vi "PowerConversion.vi"() -> ()   [LabVIEW 2017, in "HMILibrary.lvlib"]
uses:
  HMILibrary.lvlib
  <vilib>/Platform/TimedLoop/XDataNode/timing_clust.ctl
  <vilib>/Platform/TimedLoop/XDataNode/nitl_modes.ctl
  <vilib>/Platform/TimedLoop/XDataNode/wakeup.ctl
  <vilib>/platform/TimedLoop/XDataNode/XDataNode.xnode
  <vilib>/express/express arith-compare/Formula/XNode/ExpressFormulaBlockNode.xnode
  <vilib>/Platform/TimedLoop/XDataNode/XDNodeRunTimeDep.lvlib
panel:
  out "P_1":dbl
  out "T_1":dbl
  out "P_2":dbl
  out "T_2":dbl
  out "P_3":dbl
  out "T_3":dbl
  out "P_4":dbl
  out "T_4":dbl
  out "P_5":dbl
  out "T_5":dbl
  out "P_6":dbl
  out "T_6":dbl
  out "R_P_4":dbl
  out "R_T_4":dbl
  out "h_4":dbl
  out "R_P_5":dbl
  out "R_T_5":dbl
  out "h_5":dbl
  out "R_P_6":dbl
  out "R_T_6":dbl
  out "h_6":dbl
  out "R_P_1":dbl
  out "R_T_1":dbl
  out "h_1":dbl
  in  "Compression Ratio":dbl=19.6
  in  "Incoming Air Temp":dbl=298.0
  in  "HPT Expansion Ratio":dbl=3.77
  in  "Incoming Air Pressure":dbl=101325.0
  in  "LPT Expansion Ratio":dbl=5.13
  in  "Compressor Efficiency":dbl=0.7
  in  "HPT Efficiency":dbl=0.8
  in  "LPT Efficiency":dbl=0.8
  in  "HPT Work Output":dbl=1000000.0
  in  "LPT Work Output":dbl=137940000.0
  in  "Pressure Drop in HX 1st pass":dbl
  in  "Pressure Drop in HX 2nd pass":dbl
  in  "Mass Flowrate":dbl=418.0
  in  "Lower Operating Pressure":dbl=7093.0
  in  "Pinch Point Temp Difference":dbl=15.0
  in  "Turbine Efficiency":dbl=0.95
  in  "Pump Efficiency":dbl=0.95
  in  "Upper Operating Pressure":dbl=6154480.5
  in  "stop":bool
  # "Power Conversion System"
  # "Brayton Cycle"
  # "Rankine Cycle"
  # "HRSG"
  # "Compressor"
  # "HPT"
  # "LPT"
  # "ST"
  # "Primary Heat\nExchanger"
  # "Condenser"
  # "Pump"
  # "Temperatures in K\nPressures in Pa"
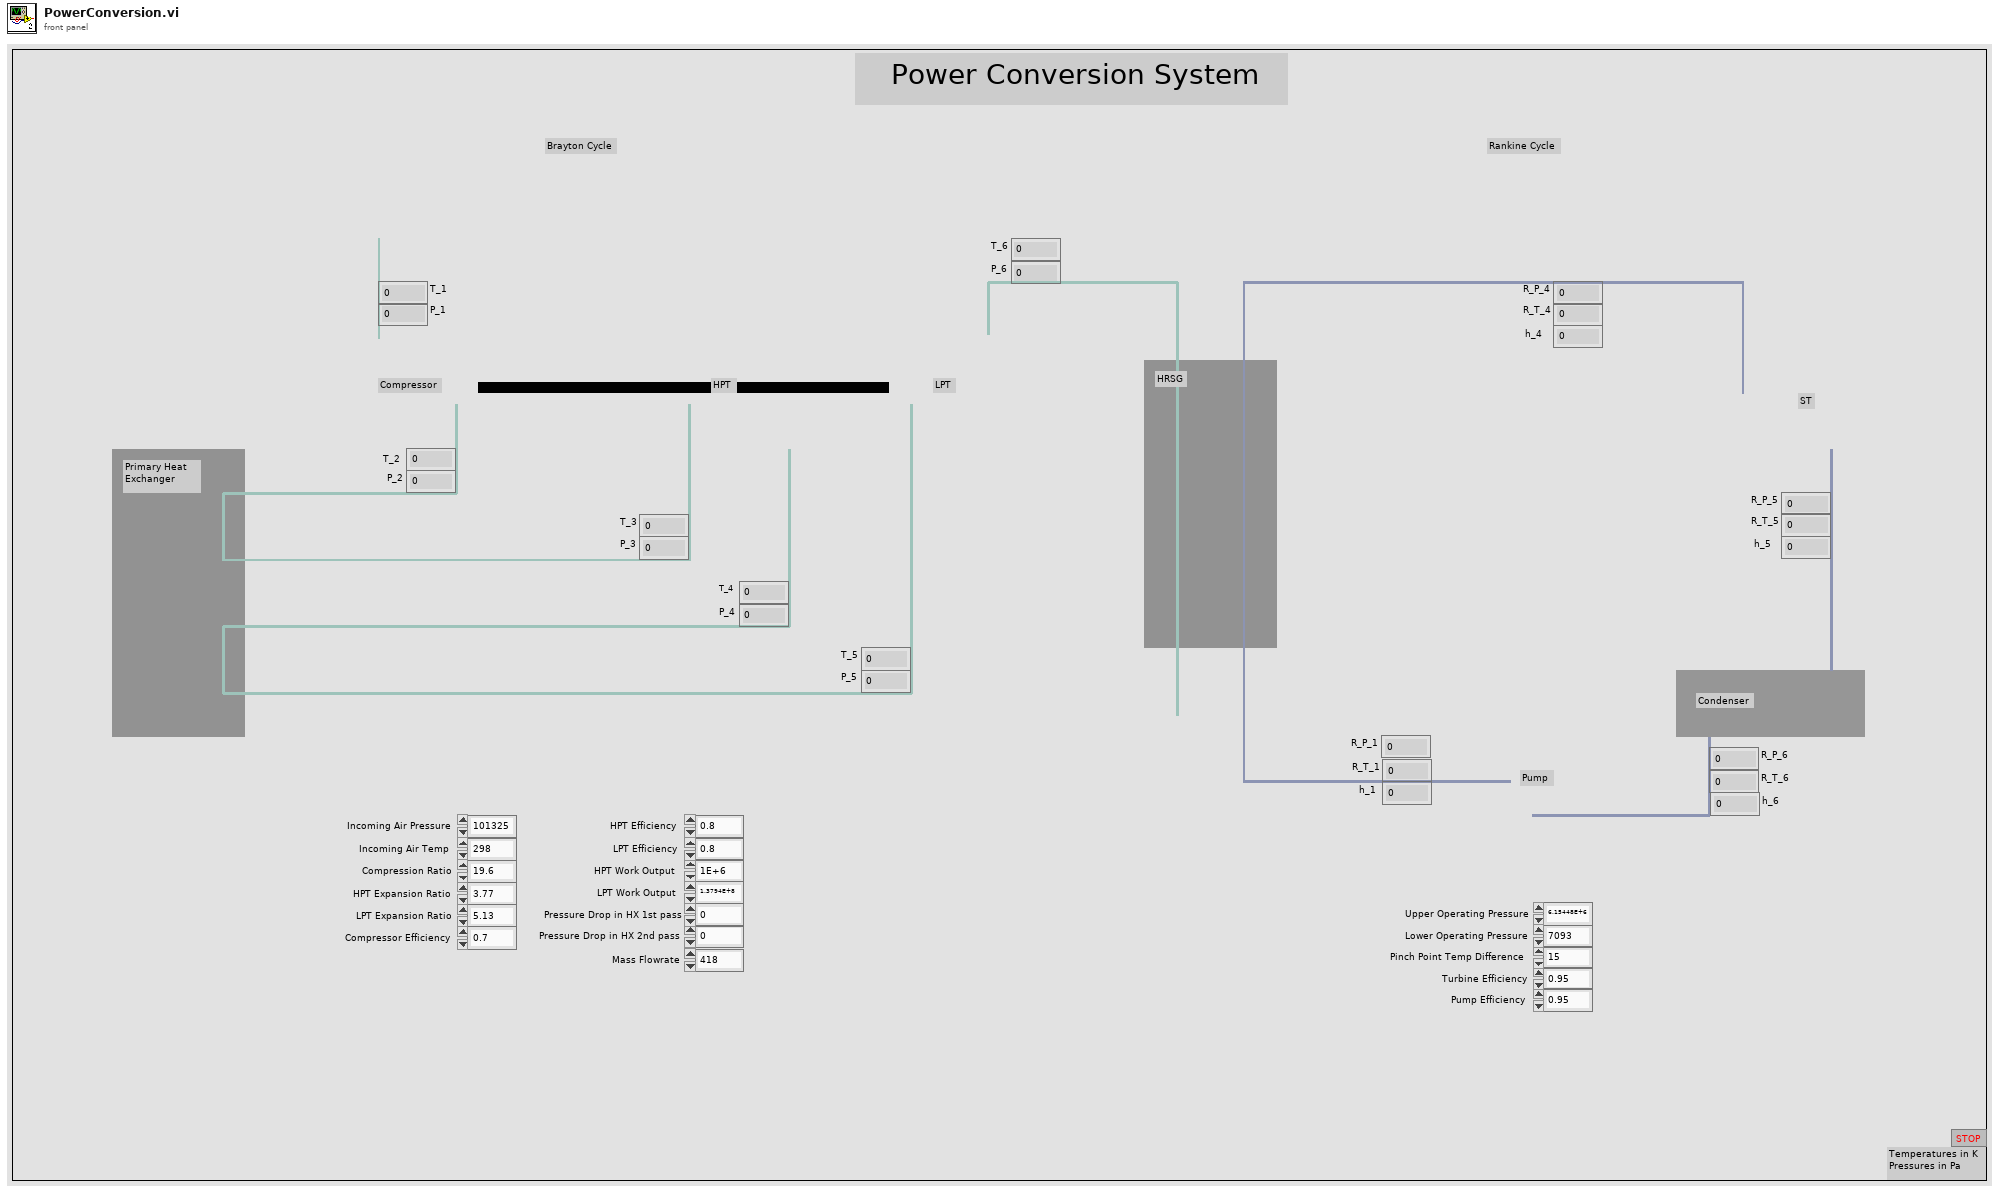
[diagram p1: front panel]
types:
  T1 = typedef "XDNodeRunTimeDep.lvlib/timing_clust.ctl" = cluster{"Expected End [f-1]":u64, "Actual End [f-1]":u64, "Finished Late? [f-1]":bool, "Expected End [i-1]":u64, "Actual End [i-1]":u64, "Finished Late? [i-1]":bool, "Expected Start [i]":u64, "Actual Start [i]":u64, "Expected Start [f]":u64, "Actual Start [f]":u64, "Source Name":string, "Structure Name":string, "Period":i64, "Deadline":i64, "Offset":i64, "Start":i64, "Priority":i32, "Timeout":i32, "Mode":T2, "Wakeup Reason":T3, "Error":errorcluster, "Source Type":string, "Secondary Source Type":string, "Global End Time":u64, "Global Start Time":u64, "Frame Duration":u64, "Iteration Duration":u64, "Assigned CPU":i32, "I/O Scan Engine Mode":u32}
  T2 = typedef "XDNodeRunTimeDep.lvlib/nitl_modes.ctl" = enum32{"No Change", "Process missed periods, maintain original phase", "Discard missed periods, maintain original phase", "Process missed periods, ignore original phase", "Discard missed periods, ignore original phase"}
  T3 = typedef "XDNodeRunTimeDep.lvlib/wakeup.ctl" = enum32{"Normal", "Aborted", "Asynchronous wakeup", "Timing source error", "Timed loop error", "Timeout"}
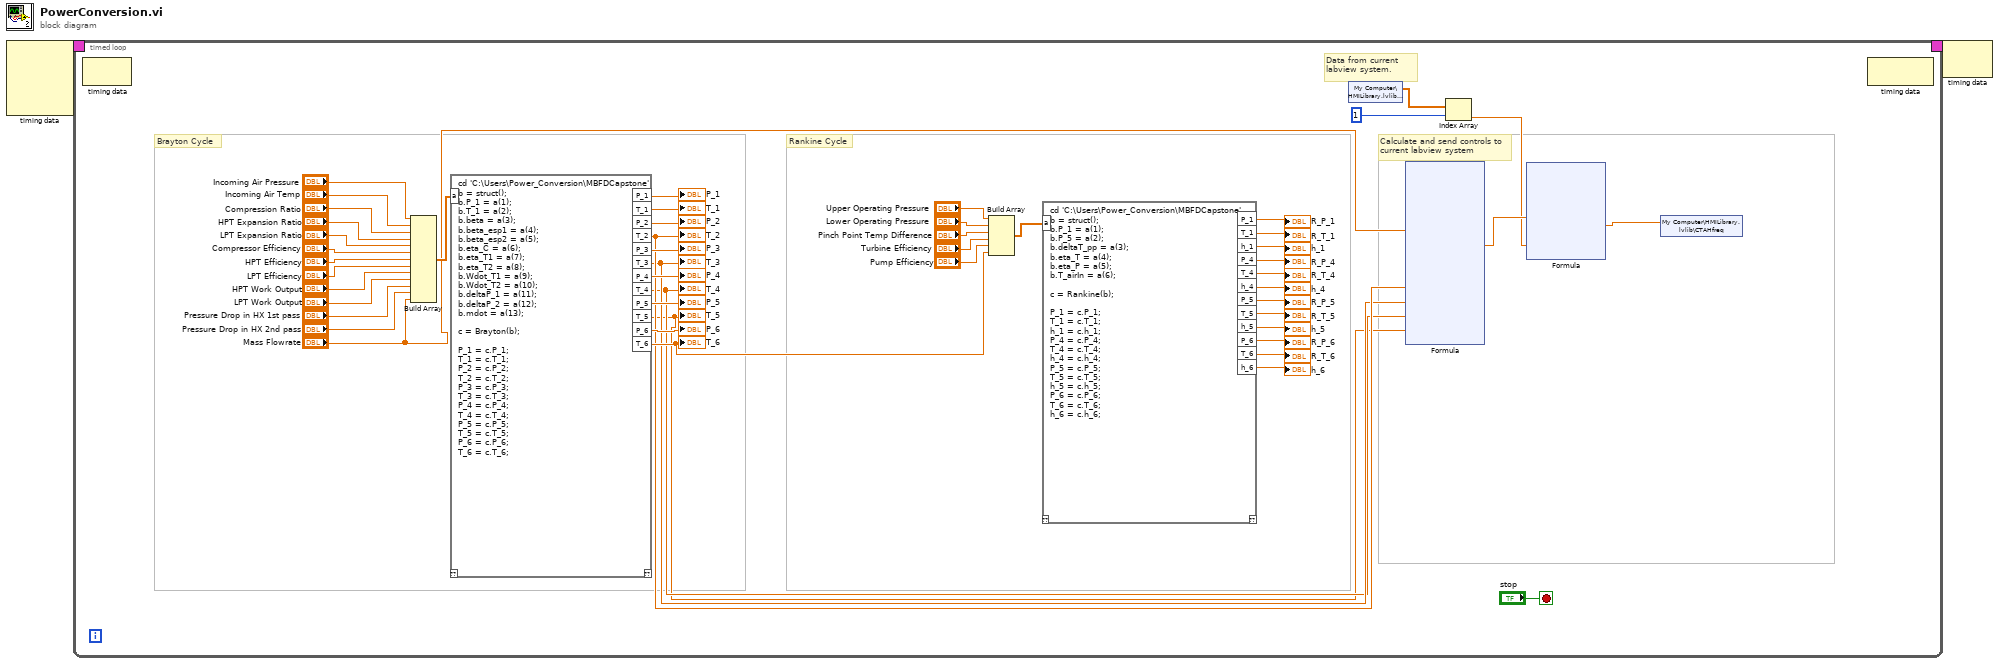
[diagram p0: block diagram]
diagram:
  n1 = node-c288() -> (w2:T1)  [unwired: 4 in]
  n2 = timed-loop {
    timing: w2 -> [_]
    timing-out: [_] -> w1
    stop <- "stop" stop-if-true
    # "Data from current labview system."
    # "Calculate and send controls to current labview system"
    # "Rankine Cycle"
    # "Brayton Cycle"
    n3 = node-c288() -> ()  [unwired: 1 in, 1 out]
    n4 = Build Array("Incoming Air Pressure", "Incoming Air Temp", "Compression Ratio", "HPT Expansion Ratio", "LPT Expansion Ratio", "Compressor Efficiency", "HPT Efficiency", "LPT Efficiency", "HPT Work Output", "LPT Work Output", "Pressure Drop in HX 1st pass", "Pressure Drop in HX 2nd pass", "Mass Flowrate") -> (w40:dbl[])
    n5 = script code="cd 'C:\\Users\\Power_Conversion\\MBFDCapstone'\nb = struct();\nb.P_1 = a(1);\nb.T_1 = a(2);\nb.beta = a(3);\nb.beta_esp1 = a(4);\nb.beta_esp2 = a(5);\nb.eta_C = a(6);\nb.eta_T1 = a(7);\nb.eta_T2 = a(8);\nb.Wdot_T1 = a(9);\nb.Wdot_T2 = a(10);\nb.deltaP_1 = a(11);\nb.deltaP_2 = a(12);\nb.mdot = a(13);\n\nc = Brayton(b);\n\nP_1 = c.P_1;\nT_1 = c.T_1;\nP_2 = c.P_2;\nT_2 = c.T_2;\nP_3 = c.P_3;\nT_3 = c.T_3;\nP_4 = c.P_4;\nT_4 = c.T_4;\nP_5 = c.P_5;\nT_5 = c.T_5;\nP_6 = c.P_6;\nT_6 = c.T_6;"("a"=w40) -> ("P_1"=→"P_1":dbl, "T_1"=→"T_1":dbl, "P_2"=→"P_2":dbl, "T_2"=w11:dbl, "P_3"=→"P_3":dbl, "T_3"=w10:dbl, "P_4"=→"P_4":dbl, "T_4"=w9:dbl, "P_5"=→"P_5":dbl, "T_5"=w8:dbl, "P_6"=→"P_6":dbl, "T_6"=w26:dbl)  [unwired: 1 in, 1 out]
    "T_2" <- w11
    "T_3" <- w10
    "T_4" <- w9
    "T_5" <- w8
    "T_6" <- w26
    n6 = Build Array("Upper Operating Pressure", "Lower Operating Pressure", "Pinch Point Temp Difference", "Turbine Efficiency", "Pump Efficiency", w26) -> (w27:dbl[])
    n7 = script code="cd 'C:\\Users\\Power_Conversion\\MBFDCapstone'\nb = struct();\nb.P_1 = a(1);\nb.P_5 = a(2);\nb.deltaT_pp = a(3);\nb.eta_T = a(4);\nb.eta_P = a(5);\nb.T_airIn = a(6);\n\nc = Rankine(b);\n\nP_1 = c.P_1;\nT_1 = c.T_1;\nh_1 = c.h_1;\nP_4 = c.P_4;\nT_4 = c.T_4;\nh_4 = c.h_4;\nP_5 = c.P_5;\nT_5 = c.T_5;\nh_5 = c.h_5;\nP_6 = c.P_6;\nT_6 = c.T_6;\nh_6 = c.h_6;"("a"=w27) -> ("P_1"=→"R_P_1":dbl, "T_1"=→"R_T_1":dbl, "h_1"=→"h_1":dbl, "P_4"=→"R_P_4":dbl, "T_4"=→"R_T_4":dbl, "h_4"=→"h_4":dbl, "P_5"=→"R_P_5":dbl, "T_5"=→"R_T_5":dbl, "h_5"=→"h_5":dbl, "P_6"=→"R_P_6":dbl, "T_6"=→"R_T_6":dbl, "h_6"=→"h_6":dbl)  [unwired: 1 in, 1 out]
    n8 = shared-variable "My Computer\\HMILibrary.lvlib\\T_n"() -> (w5:dbl[])  [unwired: 1 in, 1 out]
    n9 = xnode "Formula"("mdot"="Mass Flowrate", "T2"=w11, "T3"=w10, "T4"=w9, "T5"=w8) -> ("Result"=w7:dbl)  [unwired: 1 in, 1 out]
    n10 = Index Array(array=w5, index=1) -> (element=w4:dbl)
    n11 = xnode "Formula"("Pout"=w7, "Tin"=w4) -> ("Result"=w3:dbl)  [unwired: 1 in, 1 out]
    n12 = shared-variable "My Computer\\HMILibrary.lvlib\\CTAHfreq"(w3) -> ()  [unwired: 1 in, 1 out]
    n13 = node-c288() -> ()  [unwired: 1 in, 1 out]
  }
  n14 = node-c288(w1) -> ()  [unwired: 1 out]
